vi "Turn 90 deg.vi"(8 "error in":errorcluster, 9 "Auto Notifiers In":T1) -> (0 "error out":errorcluster, 1 "Auto Notifiers Out":T1)   [LabVIEW 2014]
uses:
  Auto Notifiers.ctl
  Main/Arms/Arm clapper state.ctl
  Main/Arms/Arm State.ctl
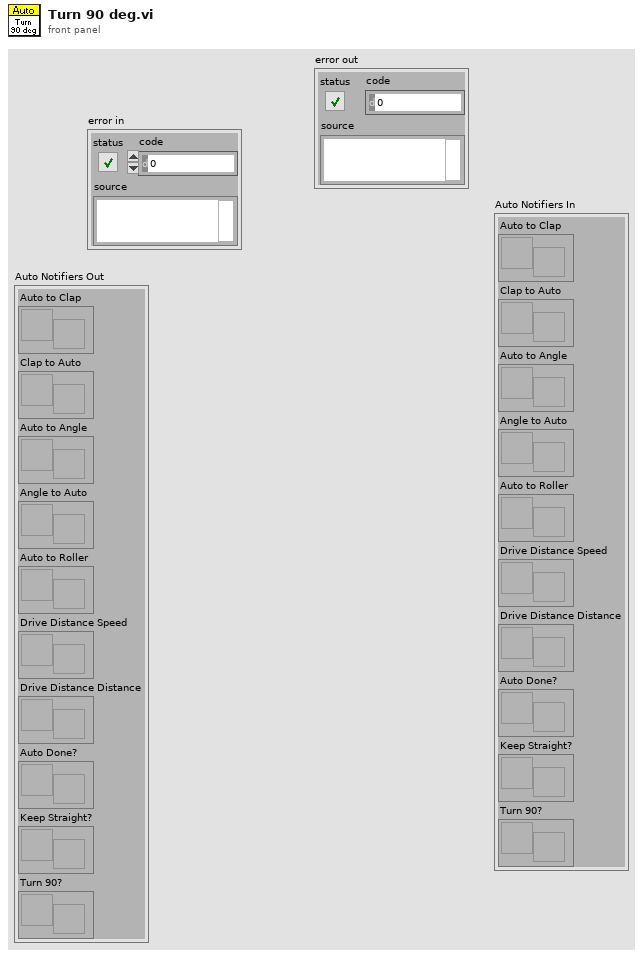
[diagram p1: front panel]
types:
  T1 = typedef "Auto Notifiers.ctl" = cluster{"Auto to Clap":refnum<notifier>, "Clap to Auto":refnum<notifier>, "Auto to Angle":refnum<notifier>, "Angle to Auto":refnum<notifier>, "Auto to Roller":refnum<notifier>, "Drive Distance Speed":refnum<notifier>, "Drive Distance Distance":refnum<notifier>, "Auto Done?":refnum<notifier>, "Keep Straight?":refnum<notifier>, "Turn 90?":refnum<notifier>}
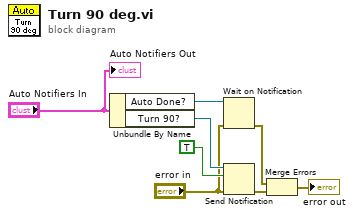
[diagram p0: block diagram]
diagram:
  n1 = Unbundle By Name("Auto Notifiers In") -> ("Auto Done?"=w6:refnum<notifier>, "Turn 90?"=w7:refnum<notifier>)
  n2 = Wait on Notification(notifier=w6, error in (no error)="error in") -> (error out=w3:errorcluster)  [unwired: 2 in, 3 out]
  n3 = Send Notification(notification=TRUE, notifier=w7, error in (no error)="error in") -> (error out=w2:errorcluster)  [unwired: 1 out]
  n4 = Merge Errors(w3, w2) -> (→"error out":errorcluster)
  "Auto Notifiers Out" <- "Auto Notifiers In"
